vi "RohitC to F.vi"() -> ()   [LabVIEW 2009]
panel:
  in  "stop":bool
  out "Farenhiet (F)":dbl(slide) scale=0.0..500.0
  in  "Celcius":dbl(slide) scale=-200.0..200.0
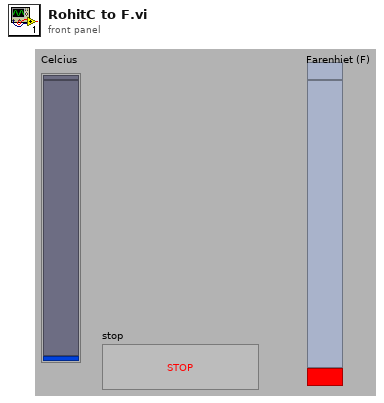
[diagram p1: front panel]
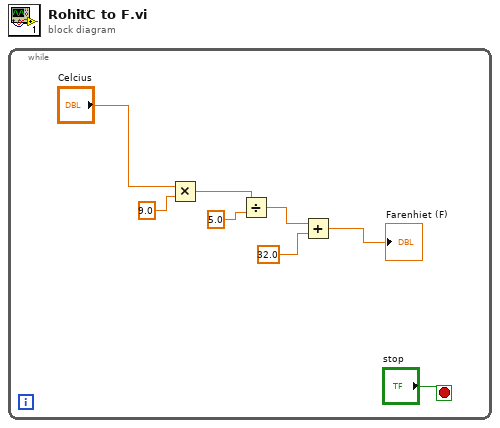
[diagram p0: block diagram]
diagram:
  n1 = while {
    stop <- "stop" stop-if-true
    n2 = Multiply(x="Celcius", y=9.0) -> (x*y=w6:dbl)
    n3 = Divide(x=w6, y=5.0) -> (x/y=w4:dbl)
    n4 = Add(x=w4, y=32.0) -> (x+y=→"Farenhiet (F)":dbl)
  }
